vi "TDTRX6-Close ActiveX.vi"(11 "error in (no error)":errorcluster) -> (15 "error out":errorcluster)   [LabVIEW 2015]
uses:
  TDT-Globals.vi
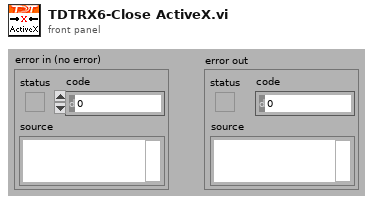
[diagram p1: front panel]
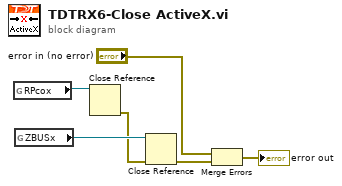
[diagram p0: block diagram]
diagram:
  n1 = global read "TDT-Globals.vi" "RPcox"() -> (w6:refnum<k7>)
  n2 = global read "TDT-Globals.vi" "ZBUSx"() -> (w5:refnum<k7>)
  n3 = Close Reference(reference=w6) -> (error out=w4:errorcluster)  [unwired: 1 in]
  n4 = Close Reference(reference=w5, error in (no error)=w4) -> (error out=w1:errorcluster)
  n5 = Merge Errors("error in (no error)", w1) -> (→"error out":errorcluster)
